vi "Motor Unwind.vi"(9 "Encoder Refnum":string="frontLeftEnc", 10 "Switch Refnum":string="My Switch RefNum", 11 "Motor Refnum":string="frontLeftRotation") -> ()   [LabVIEW 2017]
panel:
  # "Motor Unwind Autonomous Command\nFRC Team 34"
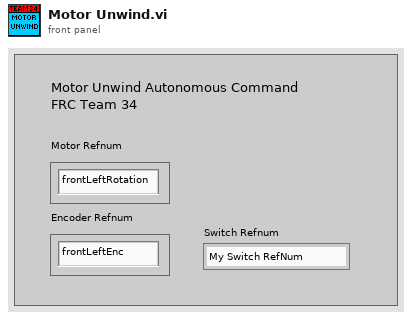
[diagram p1: front panel]
types:
  T1 = typedef "WPI_EncoderDevRef.ctl" = cluster{"DevStatus":errorcluster, "EncoderIndex":T2, "CounterIndex":T3, "DistancePerCount":dbl, "Decoding Type":T4}
  T2 = typedef "FPGA_EncoderIdx.ctl" = enum8{"Enc 0", "Enc 1", "Enc 2", "Enc 3", "Enc 4", "Enc 5", "Enc 6", "Enc 7", "Invalid"}
  T3 = typedef "FPGA_CounterCtrSystemIndex.ctl" = enum8{"Ctr 0", "Ctr 1", "Ctr 2", "Ctr 3", "Ctr 4", "Ctr 5", "Ctr 6", "Ctr 7", "Invalid"}
  T4 = typedef "WPI_EncoderType.ctl" = enum16{"1x", "2x", "4x"}
  T5 = typedef "WPI_MotorControlDeviceRef.ctl" = cluster{"DeviceStatus":errorcluster, "Type":T6, "PWM":cluster{"PWM Channel":T7, "DeadBand":T8}, "CAN":cluster{"Device Number":u8, "SetOutput VI Ref":variant, "GetOutput VI Ref":variant, "Enable VI Ref":variant, "Disable VI Ref":variant, "Data":variant}, "Invert":bool, "DIO PWM":cluster{"PWM \"Enable\" Channel":T7, "DIOChannel":T9, "PWM Rate":dbl}}
  T6 = typedef "WPI_MotorControlType.ctl" = enum16{"PWM", "CAN", "DIO PWM"}
  T7 = typedef "FPGA_DIOPWMChannel.ctl" = enum8{"PWM 0", "PWM 1", "PWM 2", "PWM 3", "PWM 4", "PWM 5", "PWM 6", "PWM 7", "PWM 8", "PWM 9", "PWM MXP 0", "PWM MXP 1", "PWM MXP 2", "PWM MXP 3", "PWM MXP 4", "PWM MXP 5", "PWM MXP 6", "PWM MXP 7", "PWM MXP 8", "PWM MXP 9", "Invalid"}
  T8 = typedef "WPI_PWMDeadband.ctl" = cluster{"Name":string, "maxPositivePwm":i32, "minPositivePwm":i32, "centerPwm":i32, "maxNegativePwm":i32, "minNegativePwm":i32, "angularRange":u16}
  T9 = typedef "FPGA_DIOChannel.ctl" = enum8{"DIO 0", "DIO 1", "DIO 2", "DIO 3", "DIO 4", "DIO 5", "DIO 6", "DIO 7", "DIO 8", "DIO 9", "DIO MXP 0", "DIO MXP 1", "DIO MXP 2", "DIO MXP 3", "DIO MXP 4", "DIO MXP 5", "DIO MXP 6", "DIO MXP 7", "DIO MXP 8", "DIO MXP 9", "DIO MXP 10", "DIO MXP 11", "DIO MXP 12", "DIO MXP 13", "DIO MXP 14", "DIO MXP 15", "SPI Port CS1", "SPI Port CS2", "SPI Port CS3", "SPI Port MISO", "SPI Port MOSI", "Invalid"}
  T10 = typedef "WPI_SwitchDevRef.ctl" = cluster{"DevStatus":errorcluster, "DIO Channel":T9, "CntIndex":T3, "Normally Closed":bool}
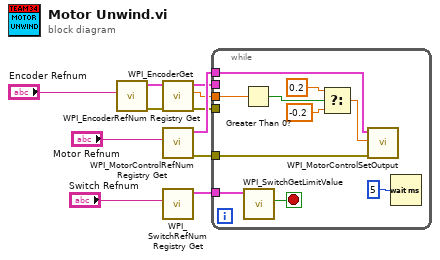
[diagram p0: block diagram]
diagram:
  n1 = call <vilib>:"WPI_EncoderRefNum Registry Get.vi"("refnum name"="Encoder Refnum") -> ("error out"=w4:errorcluster, "EncoderDevRef"=w3:T1)  [unwired: 9 in]
  n2 = call <vilib>:"WPI_EncoderGet.vi"("error in (no error)"=w4, "EncoderDevRef"=w3) -> ("error out"=w5:errorcluster, "Distance"=w7:dbl, "EncoderDevRef"=w6:T1)  [unwired: 4 in, 3 out]
  n3 = call <vilib>:"WPI_MotorControlRefNum Registry Get.vi"("refnum name"="Motor Refnum") -> ("error out"=w9:errorcluster, "MotorControlDevRef"=w8:T5)  [unwired: 9 in]
  n4 = call <vilib>:"WPI_SwitchRefNum Registry Get.vi"("refnum name"="Switch Refnum") -> ("SwitchDevRef"=w1:T10)  [unwired: 9 in, 1 out]
  n5 = while {
    tunnel: w6 -> [_]
    tunnel: w5 -> [_]
    tunnel: w7 -> [w21]
    tunnel: w8 -> [w16]
    tunnel: w9 -> [w15]
    tunnel: w1 -> [w12]
    stop <- w13 stop-if-true
    n6 = Greater Than 0?(x=w21) -> (x > 0?=w20:bool)
    n7 = call <vilib>:"WPI_SwitchGetLimitValue.vi"("SwitchDevRef"=w12) -> ("Switch Pressed"=w13:bool)  [unwired: 8 in, 2 out]
    n8 = Select(t=0.2, s=w20, f=-0.2) -> (s? t:f=w14:dbl)
    n9 = call <vilib>:"WPI_MotorControlSetOutput.vi"("error in (no error)"=w15, "Output"=w14, "MotorControlDevRef"=w16) -> ()  [unwired: 6 in, 3 out]
    n10 = Wait (ms)(milliseconds to wait=u32 5) -> ()  [unwired: 1 out]
  }
